vi "setUp.vi"(8 "error in (no error)":errorcluster, 11 "reference in":refnum<class "Transfer Group Tests.lvclass">) -> (0 "error out":errorcluster, 3 "reference out":refnum<class "Transfer Group Tests.lvclass">)   [LabVIEW 2019, in "Transfer Group Tests.lvclass"]
doc: "setUp runs prior to the test method during test execution. Use this method to initialize any object data required by your tests."
uses:
  Transfer Group Tests.lvclass
  C:/Program Files (x86)/National Instruments/LabVIEW 2019/vi.lib/addons/_JKI Toolkits/VI Tester/TestCase.llb/TestCase.lvclass
  Classes/Transfer Group/Transfer Group.lvclass
  Transfer Group Tests.lvclass/Transfer Group Tests.ctl
  <vilib>/addons/_JKI Toolkits/VI Tester/TestCase.llb/TestCase.lvclass
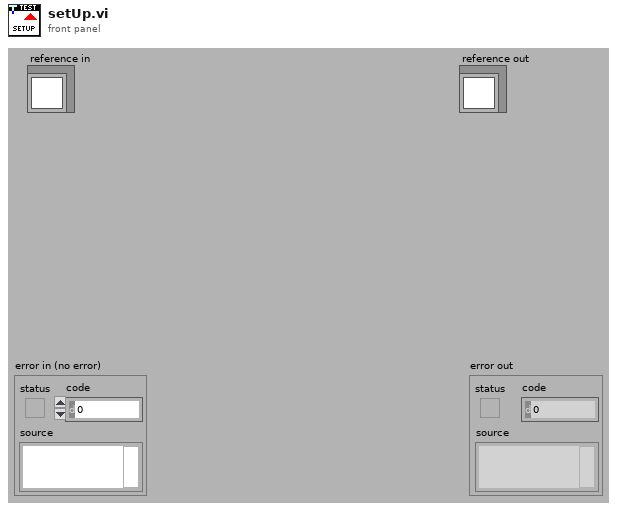
[diagram p1: front panel]
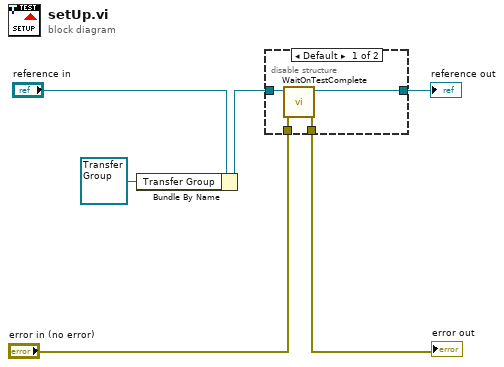
[diagram p0: block diagram]
diagram:
  n1 = Bundle By Name(cluster="reference in", "Transfer Group"=refnum<class "Transfer Group.lvclass"> refnum) -> (w2:refnum<class "Transfer Group Tests.lvclass">)
  n2 = disable-structure shown="Default" {
    disable-tunnel: "error in (no error)" -> [w10 w11]
    disable-tunnel: [w9 w11] -> w5
    disable-tunnel: [w8 w12] -> w3
    disable-tunnel: w2 -> [w7 w12]
    frame condition #0 (active) {
      n3 = call <vilib>:"WaitOnTestComplete.vi"("error in (no error)"=w10, "TestCase in"=w7) -> ("error out"=w9:errorcluster, "TestCase out"=w8:refnum<class "Transfer Group Tests.lvclass">)  [unwired: 8 in]
    }
    frame condition #1 {
    }
  }
  "error out" <- w5
  "reference out" <- w3
